vi "All Characters in a Font.vi"() -> ()   [LabVIEW 2020]
panel:
  out "Characters":string[][](array[string])
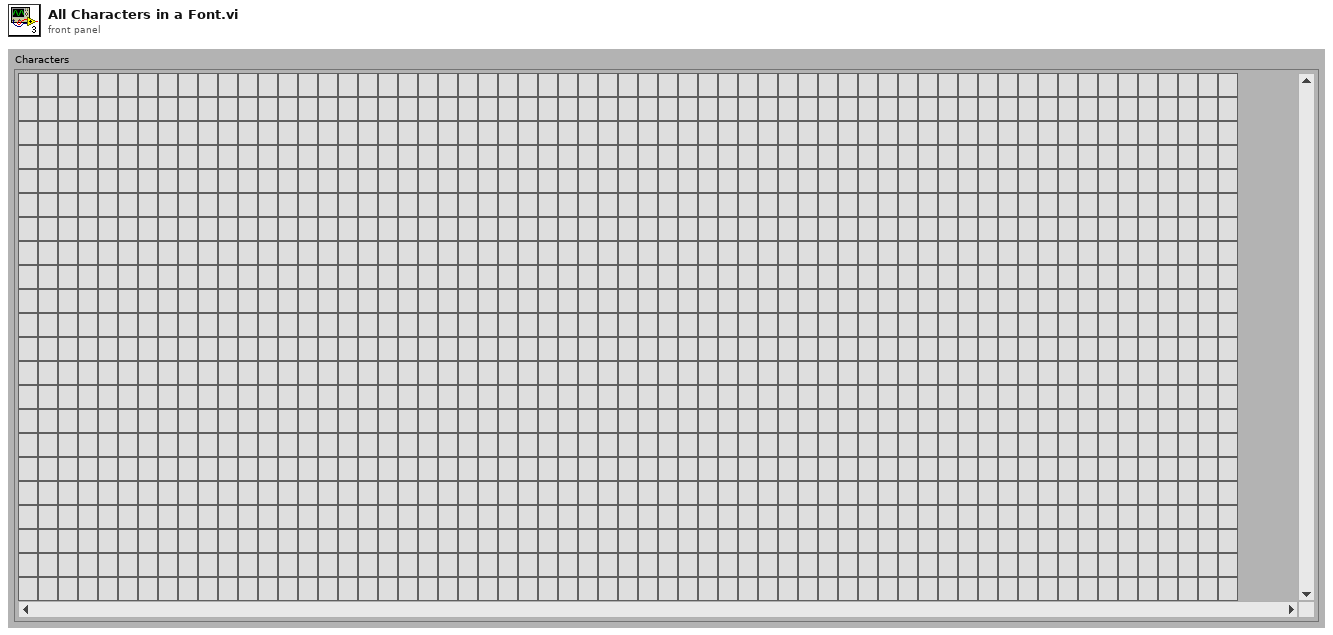
[diagram p1: front panel]
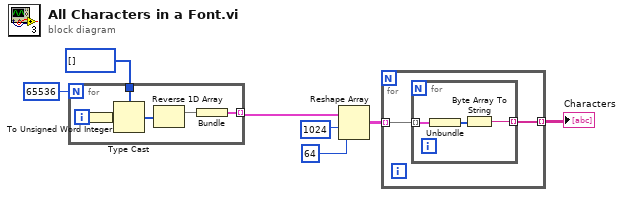
[diagram p0: block diagram]
diagram:
  n1 = for {
    N: 65536 -> [_]
    tunnel: u8[] [] -> [w12]
    tunnel: [w8] -> w5 mode=indexing
    i -> [w13]
    n2 = To Unsigned Word Integer(number=w13) -> (unsigned 16bit integer=w10:u16)
    n3 = Type Cast(type=w12, x=w10) -> (*(type *) &x=w11:u8[])
    n4 = Reverse 1D Array(array=w11) -> (reversed array=w9:u8[])
    n5 = Bundle(w9) -> (w8:cluster{u8[]})  [unwired: 1 in]
  }
  n6 = Reshape Array(w5, 1024 ("dimension size"), 64 ("dimension size")) -> (w4:cluster{u8[]}[][])
  n7 = for {
    tunnel: w4 -> [w15] mode=indexing
    tunnel: [w14] -> w3 mode=indexing
    n8 = for {
      tunnel: w15 -> [w18] mode=indexing
      tunnel: [w16] -> w14 mode=indexing
      n9 = Unbundle(w18) -> (w17:u8[])
      n10 = Byte Array To String(unsigned byte array=w17) -> (string=w16:string)
    }
  }
  "Characters" <- w3
